vi "Set Debug Flag.vi"(8 "error in":errorcluster, 10 "Debug Setting":bool) -> (0 "error out":errorcluster)   [LabVIEW 2020]
doc: "Turns the Debug global variable on or off and then saves the global variable."
uses:
  <vilib>/Utility/traverseref.llb/VI Scripting - Traverse.lvlib
  <vilib>/Utility/traverseref.llb/TRef TravTarget.ctl
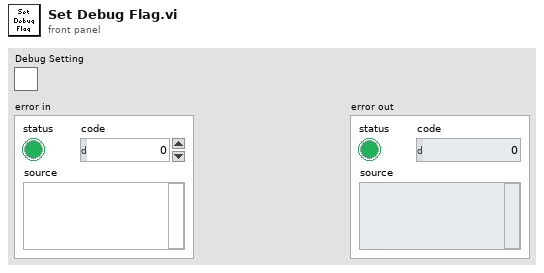
[diagram p1: front panel]
types:
  T1 = typedef "TRef TravTarget.ctl" = enum16{"FP", "BD", "Other"}
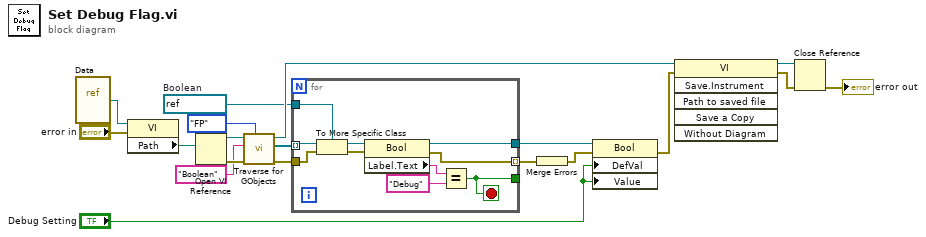
[diagram p0: block diagram]
diagram:
  w5 = refnum<vi> refnum  # Boolean
  n1 = vi-ref "Data.vi"() -> (w12:refnum<vi>)
  n2 = property class="VI"(reference=w12, error in="error in") -> ("Path"=w1:path)  [unwired: 2 out]
  n3 = Open VI Reference(vi path=w1) -> (vi reference=w8:refnum<vi>, error out=w15:errorcluster)  [unwired: 5 in]
  n4 = call <vilib>:"Traverse for GObjects.vi"("Traverse Target"=TRef_TravTarget."FP", "error in (no error)"=w15, "Class Name"="Boolean", "VI Refnum"=w8) -> ("error out"=w16:errorcluster, "References"=w4:refnum<vi>[], "dup VI Refnum"=w10:refnum<vi>)  [unwired: 4 in, 1 out]
  n5 = for {
    tunnel: w4 -> [w26] mode=indexing
    tunnel: w16 -> [w29]
    tunnel: w5 -> [w24]
    tunnel: [w27] -> w6 mode=indexing
    tunnel: [w21] -> w7
    tunnel: [w20] -> _
    stop <- w20 stop-if-true
    n6 = To More Specific Class(target class=w24, reference=w26, error in=w29) -> (specific class reference=w25:refnum<vi>, error out=w28:errorcluster)
    n7 = property class="Bool"(reference=w25, error in=w28) -> (reference out=w21:refnum<vi>, error out=w27:errorcluster, "Label.Text"=w23:string)
    n8 = Equal?(x=w23, y="Debug") -> (x = y?=w20:bool)
  }
  n9 = Merge Errors(w6) -> (w17:errorcluster)
  n10 = property class="Bool"(reference=w7, error in=w17, "DefVal"="Debug Setting", "Value"="Debug Setting") -> (error out=w18:errorcluster)  [unwired: 1 out]
  n11 = invoke class="VI" method="Save.Instrument"(reference=w10, error in=w18) -> (reference out=w11:refnum<vi>, error out=w19:errorcluster)  [unwired: 4 in, 4 out]
  n12 = Close Reference(reference=w11, error in (no error)=w19) -> (error out=→"error out":errorcluster)
